vi "Paint_Center_Mass-1.vi"(2 "error IN":errorcluster, 3 "Array of Points IN":dbl[](array[numeric]), 4 "Image IN":T1) -> (0 "error OUT":errorcluster, 1 "Image OUT":T1)   [LabVIEW 2017]
uses:
  <vilib>/vision/Image Controls.llb/IMAQ Image.ctl
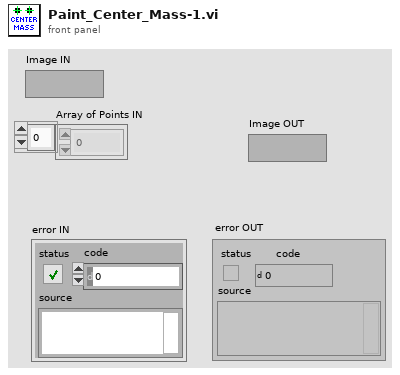
[diagram p1: front panel]
types:
  T1 = typedef "IMAQ Image.ctl" = refnum<image>
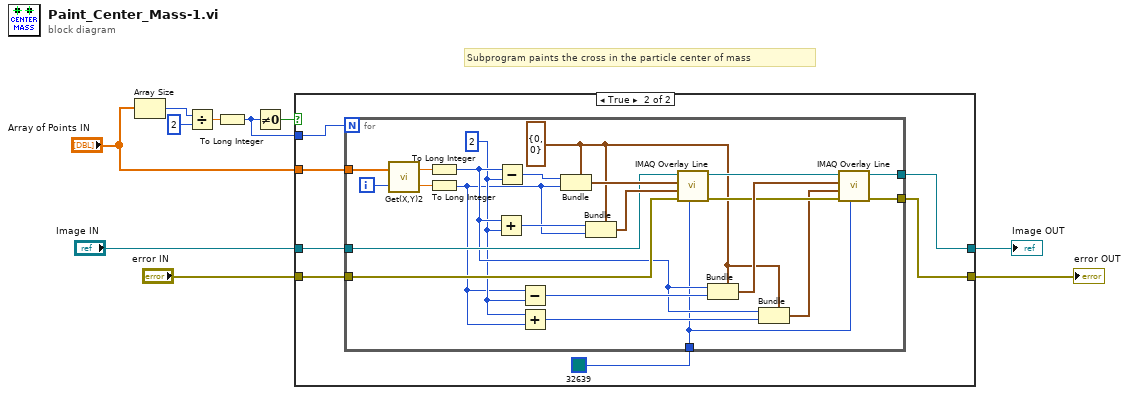
[diagram p0: block diagram]
diagram:
  # "Subprogram paints the cross in the particle center of mass"
  n1 = Array Size(array="Array of Points IN") -> (size(s)=w10:i32)
  n2 = Divide(x=w10, y=2) -> (x/y=w6:dbl)
  n3 = To Long Integer(number=w6) -> (32bit integer=w4:i32)
  n4 = Not Equal To 0?(x=w4) -> (x != 0?=w5:bool)
  n5 = case shown="True" w5 {
    tunnel: "Image IN" -> [w12 w19]
    tunnel: "Array of Points IN" -> [_ w18]
    tunnel: "error IN" -> [w11 w17]
    tunnel: w4 -> [_ w16]
    tunnel: [w12 w14] -> w2
    tunnel: [w11 w13] -> w1
    frame False {
    }
    frame True {
      n6 = for {
        N: w16 -> [_]
        tunnel: w19 -> [w34]
        tunnel: w18 -> [w42]
        tunnel: w17 -> [w33]
        tunnel: u32 32639 ("Color") -> [w22]
        tunnel: [w21] -> w14
        tunnel: [w20] -> w13
        i -> [w41]
        w28 = cluster{"X":i32, "Y":i32} {"X"=0, "Y"=0} ("Start Point")
        w26 = 2 ("y")
        n7 = call "Get(X,Y)2.vi"("[IN] index of (X,Y)"=w41, "[IN] Array coordi\nnates (X,Y) in Frame"=w42) -> ("[OUT] Y"=w39:dbl, "[OUT] X"=w40:dbl)
        n8 = To Long Integer(number=w40) -> (32bit integer=w27:i32)
        n9 = To Long Integer(number=w39) -> (32bit integer=w25:i32)
        n10 = Add(x=w27, y=w26) -> (x+y=w36:i32)
        n11 = Subtract(x=w27, y=w26) -> (x-y=w38:i32)
        n12 = Subtract(x=w25, y=w26) -> (x-y=w32:i32)
        n13 = Add(x=w26, y=w25) -> (x+y=w24:i32)
        n14 = Bundle(cluster=w28, "X"=w38, "Y"=w25) -> (w37:cluster{"X":i32, "Y":i32})
        n15 = Bundle(cluster=w28, "X"=w36, "Y"=w25) -> (w35:cluster{"X":i32, "Y":i32})
        n16 = call "IMAQ Overlay Line"("Color"=w22, "error in (no error)"=w33, "End Point"=w35, "Start Point"=w37, "Image"=w34) -> ("error out"=w29:errorcluster, "Image Out"=w30:T1)  [unwired: 5 in]
        n17 = Bundle(cluster=w28, "X"=w27, "Y"=w32) -> (w31:cluster{"X":i32, "Y":i32})
        n18 = Bundle(cluster=w28, "X"=w27, "Y"=w24) -> (w23:cluster{"X":i32, "Y":i32})
        n19 = call "IMAQ Overlay Line"("Color"=w22, "error in (no error)"=w29, "End Point"=w23, "Start Point"=w31, "Image"=w30) -> ("error out"=w20:errorcluster, "Image Out"=w21:T1)  [unwired: 5 in]
      }
    }
  }
  "Image OUT" <- w2
  "error OUT" <- w1
